vi "Actor Core.vi"(8 "error in":errorcluster, 11 "For Loop Dialog In":refnum<class "Conditional Dialog.lvclass">) -> (0 "error out":errorcluster, 3 "Actor out":refnum<class "Actor.lvclass">)   [LabVIEW 2017, in "Conditional Dialog.lvclass"]
doc: "(<B>Filename</B>: Actor Framework.lvlib:Actor.lvclass:Actor Core.vi)\n\nReceives messages to the actor, reacts to them, and initiates any error handling that may shut the actor down.\n\nDescendant classes may override this VI to append parallel tasks for the actor to complete while it handles messages. Overrides use the Call Parent Method node.\n\n<License>\nCopyright © 2017 Composed Systems, LLC | All rights reserved\nwww.composed.io\n\nAuthor: Ethan Stern <ethan.stern@composed.io>\n\nThis software is provided \"AS IS\" WITHOUT WARRANTIES, either express or implied, AND IS FOR EDUCATIONAL PURPOSES ONLY.\n</License>"
uses:
  Conditional Dialog.lvclass
  ITest Executive Builder Dialog/ITest Executive Builder Dialog.lvclass
  <vilib>/gpm_packages/@cs/mva-viewable/Source/ActorEvents/IEventAggregator/IEventAggregator.lvclass
  <vilib>/event_ctls.llb/lveventtype.ctl
  C:/Users/jonmc/Documents/Git/Test Executive Builder/Source/Test Executive Builder Dialogs/ITest Executive Builder Dialog/ITest Executive Builder Dialog.lvclass
  C:/Users/jonmc/Documents/Git/Test Executive Builder/gpm_packages/@cs/popup-viewmanager/Source/Popup ViewManager/Popup ViewManager.lvclass
  C:/Users/jonmc/Documents/Git/Test Executive Builder/gpm_packages/@cs/mva-dialogbox/source/IDialogBox/IDialogBox/IDialogBox.lvclass
  C:/Users/jonmc/Documents/Git/Test Executive Builder/gpm_packages/@cs/mva-viewable/Source/IViewable/IViewable/IViewable.lvclass
  C:/Users/jonmc/Documents/Git/Test Executive Builder/gpm_packages/@cs/mva-viewable/Source/ActorEvents/IEventAggregator/IEventAggregator.lvclass
  C:/Users/jonmc/Documents/Git/Test Executive Builder/gpm_packages/@cs/mva-core/Source/IObserver/IObserver/IObserver.lvclass
  C:/Program Files (x86)/National Instruments/LabVIEW 2017/vi.lib/ActorFramework/Actor/Actor.lvclass
  <vilib>/gpm_packages/@cs/run-time-assertions/Source/Assert Equal/Assert Equal.lvclass
  <vilib>/gpm_packages/@cs/run-time-assertions/Source/Assert Greater or Equal/Assert Greater or Equal.lvclass
  <vilib>/gpm_packages/@cs/run-time-assertions/Source/Assert Greater/Assert Greater.lvclass
  <vilib>/gpm_packages/@cs/run-time-assertions/Source/Assert Less or Equal/Assert Less or Equal.lvclass
  <vilib>/gpm_packages/@cs/run-time-assertions/Source/Assert Less/Assert Less.lvclass
  <vilib>/gpm_packages/@cs/run-time-assertions/Source/Assert Not Equal/Assert Not Equal.lvclass
  C:/Users/jonmc/Documents/Git/Test Executive Builder/gpm_packages/@cs/run-time-assertions/Source/Assert/Assert.lvclass
  <vilib>/ActorFramework/Actor/Actor.lvclass
panel:
  in  "Restore Point":bool
  in  "Variable Y":u16(ring)
  in  "Assertion":u16(ring)
  in  "Notes":string
  in  "Variable X":u16(ring)
  in  "Cancel":bool
  in  "OK":bool
  in  "Name":string
  # "Edit Conditional Statement"
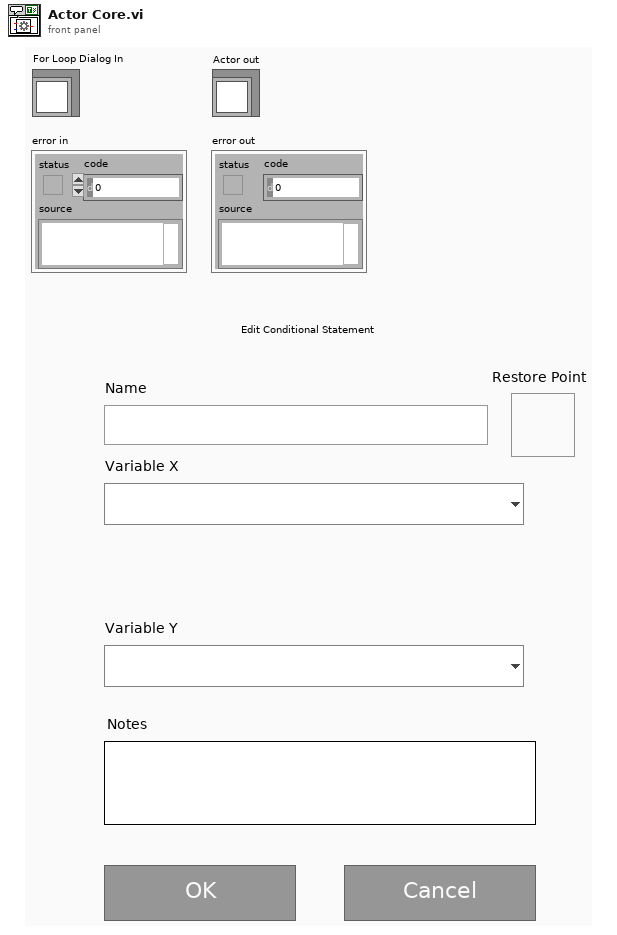
[diagram p1: front panel]
types:
  T1 = typedef "lveventtype.ctl" = enum32{"Null", "Timeout", "Annotation Menu Selection", "Annotation Menu Selection?", "App Instance Close", "App Instance Close?", "Autoscale Range Change", "Bookmark Info Change", "Cell Edit", "Cell Edit?", "Cursor Grab", "Cursor Grab?", "Cursor Menu Selection", "Cursor Menu Selection?", "Cursor Move", "Cursor Release", "Data Change", "Direction Change", "Display State Change", "Drag Ended", "Drag Enter", "Drag Leave", "Drag Over", "Drag Source Update", "Drag Starting", "Drag Starting?", "Drop", "Exec State Change", "Key Down", "Key Down?", "Key Repeat", "Key Repeat?", "Key Up", "Listbox Double Click", "Menu Activation?", "Menu Selection (App)", "Menu Selection? (App)", "Menu Selection (User)", "Mouse Down", "Mouse Down?", "Mouse Enter", "Mouse Leave", "Mouse Move", "Mouse Up", "Mouse Wheel", "NI Security User Change (App)", "Pane Size", "Panel Close", "Panel Close?", "Panel Resize", "Plot Attribute Change", "Scale Range Change", "Shortcut Menu Activation?", "Shortcut Menu Selection (App)", "Shortcut Menu Selection? (App)", "Shortcut Menu Selection (User)", "Tree Double Click", "Tree Drag", "Tree Drag?", "Tree Drop", "Tree Drop?", "Tree Item Close", "Tree Item Close?", "Tree Item Open", "Tree Item Open?", "User Event", "Value Change"}
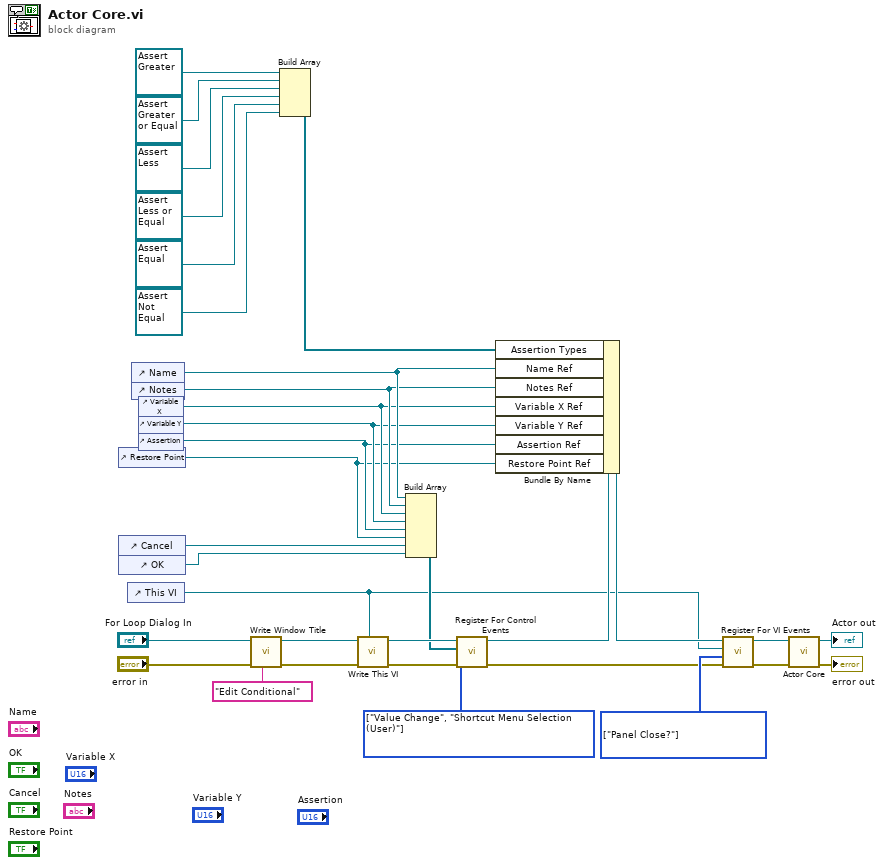
[diagram p0: block diagram]
diagram:
  w21 = T1[] [enum."Panel Close?"] items=["Null", "Timeout", "Annotation Menu Selection", "Annotation Menu Selection?", "App Instance Close", "App Instance Close?", "Autoscale Range Change", "Bookmark Info Change", "Cell Edit", "Cell Edit?", "Cursor Grab", "Cursor Grab?", "Cursor Menu Selection", "Cursor Menu Selection?", "Cursor Move", "Cursor Release", "Data Change", "Direction Change", "Display State Change", "Drag Ended", "Drag Enter", "Drag Leave", "Drag Over", "Drag Source Update", "Drag Starting", "Drag Starting?", "Drop", "Exec State Change", "Key Down", "Key Down?", "Key Repeat", "Key Repeat?", "Key Up", "Listbox Double Click", "Menu Activation?", "Menu Selection (App)", "Menu Selection? (App)", "Menu Selection (User)", "Mouse Down", "Mouse Down?", "Mouse Enter", "Mouse Leave", "Mouse Move", "Mouse Up", "Mouse Wheel", "NI Security User Change (App)", "Pane Size", "Panel Close", "Panel Close?", "Panel Resize", "Plot Attribute Change", "Scale Range Change", "Shortcut Menu Activation?", "Shortcut Menu Selection (App)", "Shortcut Menu Selection? (App)", "Shortcut Menu Selection (User)", "Tree Double Click", "Tree Drag", "Tree Drag?", "Tree Drop", "Tree Drop?", "Tree Item Close", "Tree Item Close?", "Tree Item Open", "Tree Item Open?", "User Event", "Value Change"] ("Registration Types")
  w26 = T1[] [enum."Value Change", enum."Shortcut Menu Selection (User)"] items=["Null", "Timeout", "Annotation Menu Selection", "Annotation Menu Selection?", "App Instance Close", "App Instance Close?", "Autoscale Range Change", "Bookmark Info Change", "Cell Edit", "Cell Edit?", "Cursor Grab", "Cursor Grab?", "Cursor Menu Selection", "Cursor Menu Selection?", "Cursor Move", "Cursor Release", "Data Change", "Direction Change", "Display State Change", "Drag Ended", "Drag Enter", "Drag Leave", "Drag Over", "Drag Source Update", "Drag Starting", "Drag Starting?", "Drop", "Exec State Change", "Key Down", "Key Down?", "Key Repeat", "Key Repeat?", "Key Up", "Listbox Double Click", "Menu Activation?", "Menu Selection (App)", "Menu Selection? (App)", "Menu Selection (User)", "Mouse Down", "Mouse Down?", "Mouse Enter", "Mouse Leave", "Mouse Move", "Mouse Up", "Mouse Wheel", "NI Security User Change (App)", "Pane Size", "Panel Close", "Panel Close?", "Panel Resize", "Plot Attribute Change", "Scale Range Change", "Shortcut Menu Activation?", "Shortcut Menu Selection (App)", "Shortcut Menu Selection? (App)", "Shortcut Menu Selection (User)", "Tree Double Click", "Tree Drag", "Tree Drag?", "Tree Drop", "Tree Drop?", "Tree Item Close", "Tree Item Close?", "Tree Item Open", "Tree Item Open?", "User Event", "Value Change"] ("Registration Types")
  n1 = control-ref of="Restore Point"() -> (w8:refnum<vi>)
  n2 = control-ref of="Cancel"() -> (w25:refnum<vi>)
  n3 = control-ref of="OK"() -> (w24:refnum<vi>)
  n4 = control-ref of="This VI"() -> (w16:refnum<vi>)
  n5 = control-ref of="Name"() -> (w23:refnum<vi>)
  n6 = control-ref of="Notes"() -> (w12:refnum<vi>)
  n7 = control-ref of="Variable X"() -> (w11:refnum<vi>)
  n8 = control-ref of="Variable Y"() -> (w10:refnum<vi>)
  n9 = control-ref of="Assertion"() -> (w9:refnum<vi>)
  n10 = call "Write Window Title.vi"("Window Title"="Edit Conditional", "ITest Executive Builder Dialog in"="For Loop Dialog In") -> ("ITest Executive Builder Dialog out"=w14:refnum<class "Conditional Dialog.lvclass">)  [unwired: 9 in]
  n11 = Build Array(refnum<class "Assert Greater.lvclass"> refnum ("Run Time Assertions.lvlib:Assert Greater.lvclass"), refnum<class "Assert Greater or Equal.lvclass"> refnum ("Run Time Assertions.lvlib:Assert Greater or Equal.lvclass"), refnum<class "Assert Less.lvclass"> refnum ("Run Time Assertions.lvlib:Assert Less.lvclass"), refnum<class "Assert Less or Equal.lvclass"> refnum ("Run Time Assertions.lvlib:Assert Less or Equal.lvclass"), refnum<class "Assert Equal.lvclass"> refnum ("Run Time Assertions.lvlib:Assert Equal.lvclass"), refnum<class "Assert Not Equal.lvclass"> refnum ("Run Time Assertions.lvlib:Assert Not Equal.lvclass")) -> (w1:refnum<class "Assert.lvclass">[])
  n12 = call "Write This VI.vi"("This VI"=w16, "ITest Executive Builder Dialog in"=w14) -> ("ITest Executive Builder Dialog out"=w28:refnum<class "Conditional Dialog.lvclass">)  [unwired: 9 in]
  n13 = Build Array(w23, w12, w11, w10, w9, w8, w25, w24) -> (w22:refnum<vi>[])
  n14 = call <vilib>:"Register For Control Events.vi"("error in (no error)"="error in", "Registration Types"=w26, "Control Refnums"=w22, "IEventAggregator In"=w28) -> ("error out"=w20:errorcluster, "IEventAggregator Out"=w27:refnum<class "Conditional Dialog.lvclass">)  [unwired: 6 in]
  n15 = Bundle By Name(cluster=w27, "Assertion Types"=w1, "Name Ref"=w23, "Notes Ref"=w12, "Variable X Ref"=w11, "Variable Y Ref"=w10, "Assertion Ref"=w9, "Restore Point Ref"=w8) -> (w18:refnum<class "Conditional Dialog.lvclass">)
  n16 = call <vilib>:"Register For VI Events.vi"("error in (no error)"=w20, "Registration Types"=w21, "VI Refnum"=w16, "IEventAggregator In"=w18) -> ("error out"=w19:errorcluster, "IEventAggregator Out"=w17:refnum<class "Conditional Dialog.lvclass">)  [unwired: 6 in]
  n17 = call-parent "Actor Core.vi"("error in"=w19, "ITest Executive Builder Dialog In"=w17) -> ("error out"=→"error out":errorcluster, "Actor out"=→"Actor out":refnum<class "Actor.lvclass">)  [unwired: 8 in]
